vi "Depen YAML.vi"(8 "error in (no error)":errorcluster, 9 "Level":u32, 10 "YAML String":string, 11 "Data in":variant) -> (0 "error out":errorcluster, 2 "Remaining String":string, 3 "Data out":variant)   [LabVIEW 2015, in "YAML Parser.lvclass"]
uses:
  YAML Parser.lvclass
  <vilib>/regexp/Match Regular Expression.xnode
panel:
  out "Index":u32
  out "Label":string
  out "Value":string
  out "whole match":string
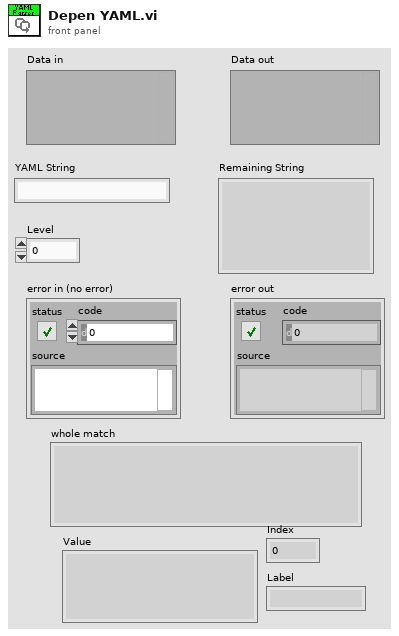
[diagram p1: front panel]
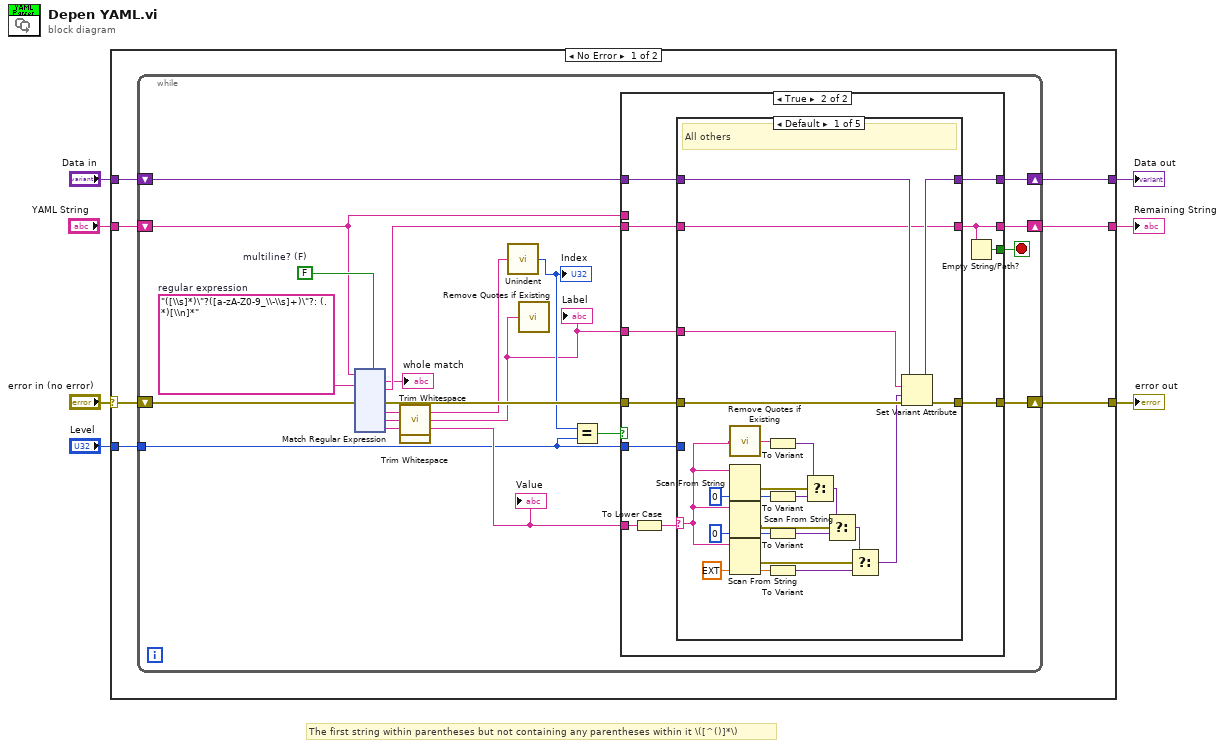
[diagram p0: block diagram]
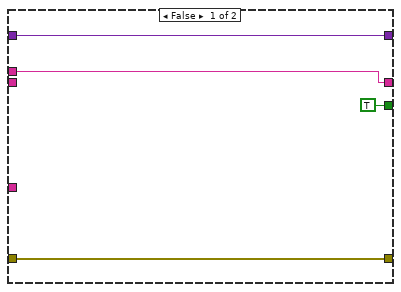
[diagram p2: hidden frame]
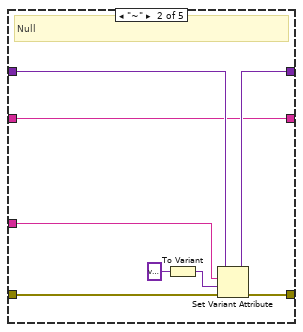
[diagram p3: hidden frame]
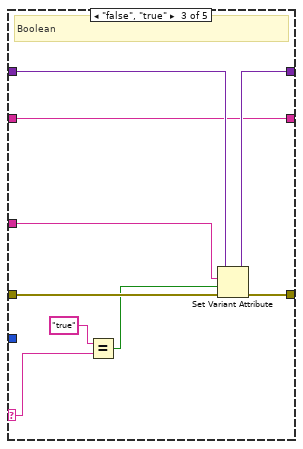
[diagram p4: hidden frame]
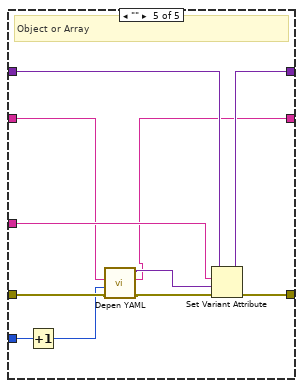
[diagram p6: hidden frame]
diagram:
  # "The first string within parentheses but not containing any parentheses within it \\([^()]*\\)"
  n1 = case shown="No Error" "error in (no error)" {
    selector: "error in (no error)" -> [w14 w224]
    tunnel: [w11 w224] -> w6
    tunnel: "Data in" -> [w12 w223]
    tunnel: "Level" -> [w8 _]
    tunnel: "YAML String" -> [w13 _]
    tunnel: [w10 w223] -> w2
    tunnel: [w9 _] -> w1
    frame No Error {
      n2 = while {
        shift-right: [w26] -> w11
        shift-left: w14 -> [w34]
        shift-right: [w25] -> w10
        shift-left: w12 -> [w28]
        shift-right: [w22] -> w9
        shift-left: w13 -> [w19]
        tunnel: w8 -> [w21]
        stop <- w24 stop-if-true
        w30 = FALSE  # multiline? (F)
        w33 = "([\\s]*)\"?([a-zA-Z0-9_\\-\\s]+)\"?: (.*)[\\n]*"  # regular expression
        n3 = xnode "Match Regular Expression"("input string"=w19, "regular expression"=w33, "error in"=w34, "multiline? (F)"=w30) -> ("whole match"=→"whole match":string, "after match"=w23:string, "error out"=w27:errorcluster, "submatch 1"=w17:string, "submatch 2"=w32:string, "submatch 3"=w31:string)  [unwired: 2 in, 2 out]
        n4 = call <vilib>:"Trim Whitespace.vi"("string"=w32) -> ("trimmed string"=w15:string)  [unwired: 1 in]
        "Label" <- w15
        n5 = call <vilib>:"Trim Whitespace.vi"("string"=w31) -> ("trimmed string"=w29:string)  [unwired: 1 in]
        "Value" <- w29
        n6 = call "Unindent.vi"("Line String"=w17) -> ("Index"=w16:u32)
        "Index" <- w16
        n7 = call "Remove Quotes if Existing.vi"("String"=w15) -> ()  [unwired: 1 out]
        n8 = Equal?(x=w16, y=w21) -> (x = y?=w20:bool)
        n9 = case shown="True" w20 {
          tunnel: w29 -> [_ w49]
          tunnel: w28 -> [w36 w47]
          tunnel: w27 -> [w35 w46]
          tunnel: [w35 w45] -> w26
          tunnel: [w36 w44] -> w25
          tunnel: w15 -> [_ w43]
          tunnel: [TRUE w42] -> w24
          tunnel: w23 -> [_ w41]
          tunnel: [w37 w40] -> w22
          tunnel: w21 -> [_ w39]
          tunnel: w19 -> [w37 _]
          frame False {
          }
          frame True {
            n10 = To Lower Case(string=w49) -> (all lower case string=w48:string)
            n11 = case shown="Default" w48 {
              selector: w48 -> [w51 _ w85 _ _]
              tunnel: w47 -> [w68 w79 w88 w93 w103]
              tunnel: w46 -> [w69 w81 w90 w92 w98]
              tunnel: [w70 w80 w89 w92 w104] -> w45
              tunnel: [w67 w78 w87 w93 w102] -> w44
              tunnel: w43 -> [w66 w77 w86 _ w101]
              tunnel: w41 -> [w52 w74 w82 w91 w97]
              tunnel: [w52 w74 w82 w91 w94] -> w40
              tunnel: w39 -> [_ _ _ _ w100]
              frame Default {
                # "All others"
                n12 = call "Remove Quotes if Existing.vi"("String"=w51) -> ("String out"=w50:string)
                n13 = Scan From String(input string=w51, default 1=i64 0) -> (error out=w62:errorcluster, output 1=w65:i64)  [unwired: 3 in, 2 out]
                n14 = Scan From String(input string=w51, default 1=u64 0) -> (error out=w59:errorcluster, output 1=w63:u64)  [unwired: 3 in, 2 out]
                n15 = Scan From String(input string=w51, default 1=ext 0.0) -> (error out=w57:errorcluster, output 1=w64:ext)  [unwired: 3 in, 2 out]
                n16 = To Variant(anything=w50) -> (Variant=w60:variant)
                n17 = To Variant(anything=w65) -> (Variant=w61:variant)
                n18 = To Variant(anything=w63) -> (Variant=w58:variant)
                n19 = To Variant(anything=w64) -> (Variant=w56:variant)
                n20 = Select(t=w60, s=w62, f=w61) -> (s? t:f=w55:variant)
                n21 = Select(t=w55, s=w59, f=w58) -> (s? t:f=w54:variant)
                n22 = Select(t=w54, s=w57, f=w56) -> (s? t:f=w53:variant)
                n23 = Set Variant Attribute(Variant=w68, name=w66, value=w53, error in=w69) -> (Variant out=w67:variant, error out=w70:errorcluster)  [unwired: 1 out]
              }
              frame "~" {
                # "Null"
                n24 = To Variant(anything=variant) -> (Variant=w75:variant)
                n25 = Set Variant Attribute(Variant=w79, name=w77, value=w75, error in=w81) -> (Variant out=w78:variant, error out=w80:errorcluster)  [unwired: 1 out]
              }
              frame "false", "true" {
                # "Boolean"
                n26 = Equal?(x="true", y=w85) -> (x = y?=w83:bool)
                n27 = Set Variant Attribute(Variant=w88, name=w86, value=w83, error in=w90) -> (Variant out=w87:variant, error out=w89:errorcluster)  [unwired: 1 out]
              }
              frame "|" {
                # "Multilines string"
              }
              frame "" {
                # "Object or Array"
                n28 = Increment(x=w100) -> (x+1=w96:u32)
                n29 = call "Depen YAML.vi"("error in (no error)"=w98, "Level"=w96, "YAML String"=w97) -> ("error out"=w99:errorcluster, "Remaining String"=w94:string, "Data out"=w95:variant)  [unwired: 6 in]
                n30 = Set Variant Attribute(Variant=w103, name=w101, value=w95, error in=w99) -> (Variant out=w102:variant, error out=w104:errorcluster)  [unwired: 1 out]
              }
            }
            n31 = Empty String/Path?(string/path=w40) -> (empty?=w42:bool)
          }
        }
      }
    }
    frame Error {
    }
  }
  "error out" <- w6
  "Data out" <- w2
  "Remaining String" <- w1
